vi "OpenImageFromFile.vi"(11 "File Path":path) -> (0 "error out":errorcluster, 3 "Image":T1(plugin-control))   [LabVIEW 2019]
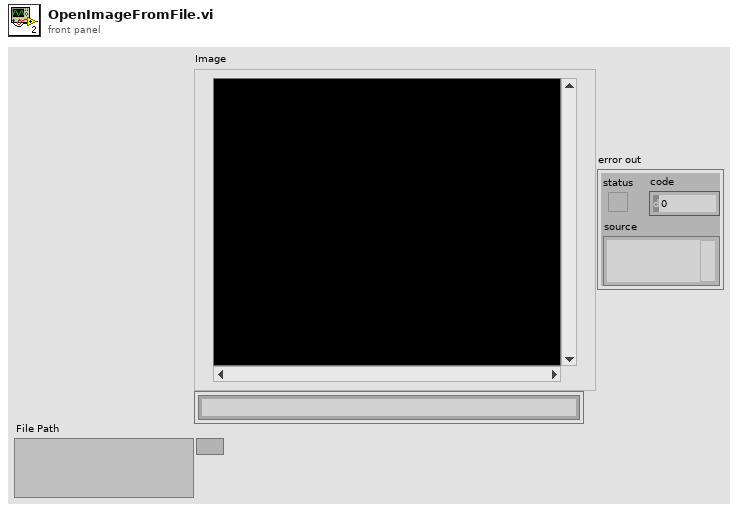
[diagram p1: front panel]
types:
  T1 = typedef "IMAQ Image.ctl" = refnum<image>
  T2 = typedef "Image Type" = u32
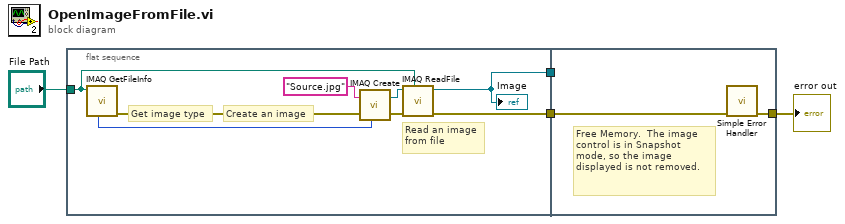
[diagram p0: block diagram]
diagram:
  n1 = flat-sequence {
    tunnel: [w7] -> w4
    tunnel: [w5] -> w3
    tunnel: "File Path" -> [w6]
    tunnel: w4 -> [w13]
    tunnel: w3 -> [_]
    tunnel: [w14] -> w2
    frame #0 {
      # "Get image type"
      # "Read an image\nfrom file"
      # "Create an image"
      n2 = call "IMAQ GetFileInfo"("File Path"=w6) -> ("error out"=w9:errorcluster, "Image Type"=w10:T2)  [unwired: 1 in, 8 out]
      n3 = call "IMAQ Create"("Image Name"="Source.jpg", "Image Type"=w10, "error in (no error)"=w9) -> ("New Image"=w11:T1, "error out"=w12:errorcluster)  [unwired: 1 in, 1 out]
      n4 = call "IMAQ ReadFile"("File Path"=w6, "error in (no error)"=w12, "Image"=w11) -> ("error out"=w7:errorcluster, "Image Out"=w5:T1)  [unwired: 2 in, 5 out]
      "Image" <- w5
    }
    frame #1 {
      # "Free Memory.  The image control is in Snapshot mode, so the image displayed is not removed."
      n5 = call <vilib>:"Simple Error Handler.vi"("error in (no error)"=w13) -> ("error out"=w14:errorcluster)  [unwired: 1 in, 7 out]
    }
  }
  "error out" <- w2
